vi "BallShear_BallShear_2.vi"(8 "Check":bool, 10 "Speed":dbl=2.0, 11 "Selected Balls":dbl[][](array[numeric])) -> (0 "Ready":bool, 2 "Waveform Stack":cluster{"Waveform Chart":dbl[]}[](array[cluster]) caption="Array of clusters, each containing one waveform chart")   [LabVIEW 2013]
panel:
  out "Status":string
  out "y":dbl
  out "x":dbl
  out "Selected Balls 2":dbl[](array[numeric])
  out "Z AFTER JOGGING":dbl
  in  "Waveform Chart":dbl(graph)
  out "Z Val":dbl
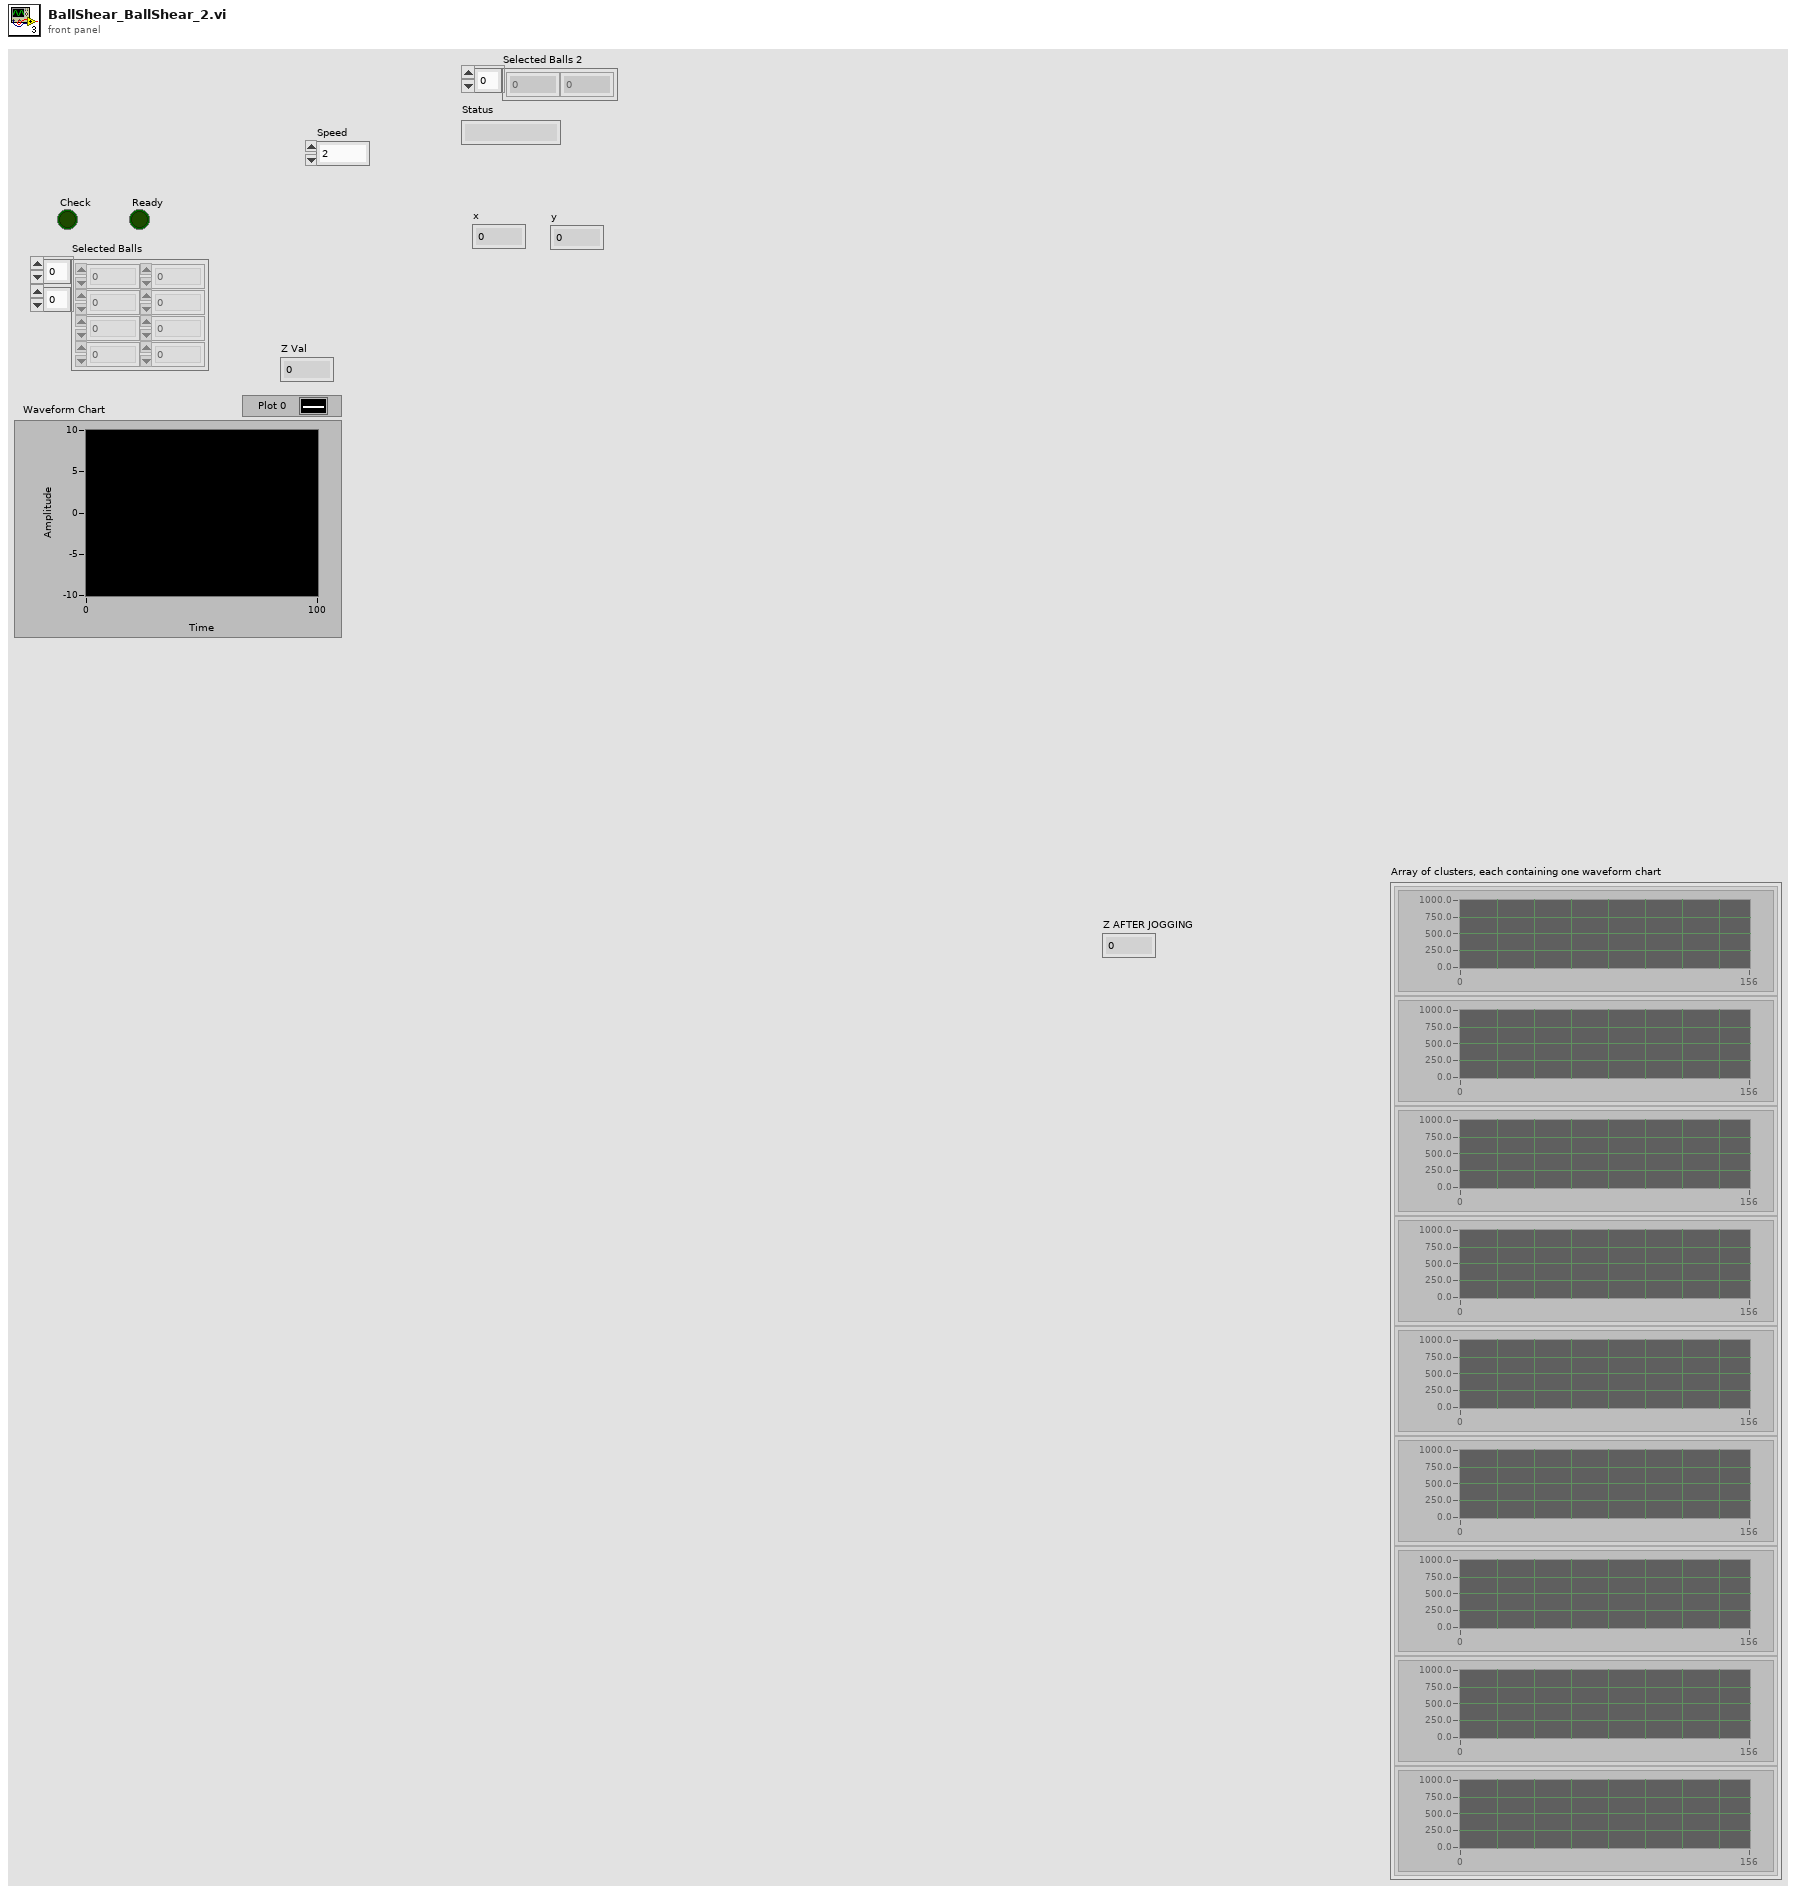
[diagram p1: front panel]
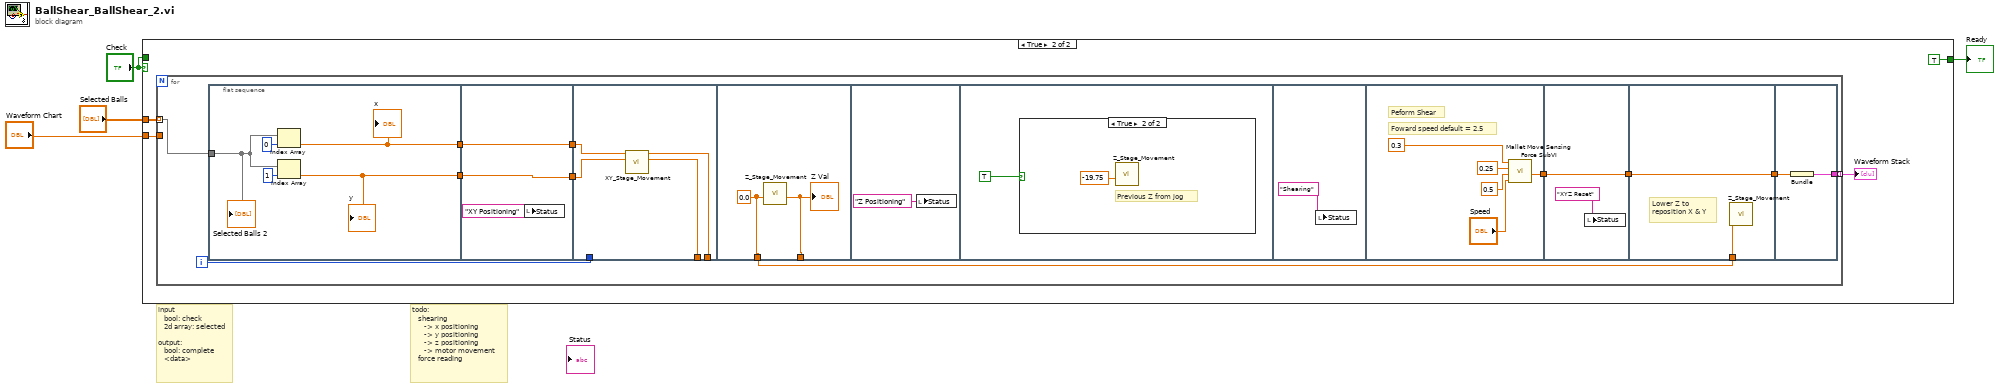
[diagram p0: block diagram]
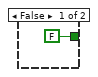
[diagram p2: hidden frame]
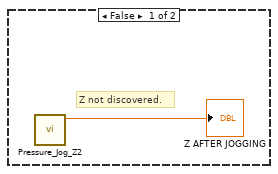
[diagram p3: hidden frame]
diagram:
  # "todo:\n   shearing\n      -> x positioning\n      -> y positioning\n      -> z positioning\n      -> motor movement\n   force reading"
  # "input\n   bool: check\n   2d array: selected\n\noutput:\n   bool: complete\n   <data>"
  n1 = case shown="True" "Check" {
    tunnel: "Check" -> [_ _]
    tunnel: [FALSE ("Power") TRUE ("Power")] -> w3
    tunnel: "Selected Balls" -> [_ w8]
    tunnel: "Waveform Chart" -> [_ w7]
    frame False {
    }
    frame True {
      n2 = for {
        tunnel: w8 -> [w16] mode=indexing
        tunnel: w7 -> [_]
        tunnel: [w19] -> w6 mode=indexing
        i -> [w20]
        n3 = flat-sequence {
          tunnel: w16 -> [w23]
          tunnel: [w22] -> w15
          tunnel: [w21] -> w13
          tunnel: w15 -> [w28]
          tunnel: [w28] -> w14
          tunnel: w13 -> [w27]
          tunnel: [w27] -> w12
          tunnel: w20 -> [_]
          tunnel: [w32] -> _
          tunnel: [w31] -> _
          tunnel: w14 -> [w30]
          tunnel: w12 -> [w29]
          tunnel: [w34] -> _
          tunnel: [w33] -> w17
          tunnel: [w40] -> w11
          tunnel: w11 -> [w46]
          tunnel: [w46] -> w10
          tunnel: w10 -> [w48]
          tunnel: [w48] -> w18
          tunnel: w17 -> [w47]
          tunnel: [w50] -> w19
          tunnel: w18 -> [w49]
          frame #0 {
            n4 = Index Array(array=w23, index=0) -> (element=w22:dbl)
            "x" <- w22
            n5 = Index Array(array=w23, index=1) -> (element=w21:dbl)
            "y" <- w21
            "Selected Balls 2" <- w23
          }
          frame #1 {
            n6 = local write "Status"("XY Positioning" ("Status")) -> ()
          }
          frame #2 {
            n7 = call "XY_Stage_Movement.vi"("Y Input"=w29, "X Input"=w30) -> ("Current Y Position"=w31:sgl, "Current X Position"=w32:sgl)  [unwired: 8 in]
          }
          frame #3 {
            w33 = 0.0 ("Z Input")
            n8 = call "Z_Stage_Movement.vi"("Z Input"=w33) -> ("Current Z Position"=w34:sgl)  [unwired: 10 in]
            "Z Val" <- w34
          }
          frame #4 {
            n9 = local write "Status"("Z Positioning" ("Status")) -> ()
          }
          frame #5 {
            n10 = case shown="True" TRUE {
              frame False {
                # "Z not discovered."
                n11 = call "Pressure_Jog_Z2.vi"() -> ("current Z"=→"Z AFTER JOGGING":sgl)  [unwired: 11 in]
              }
              frame True {
                # "Previous Z from jog"
                n12 = call "Z_Stage_Movement.vi"("Z Input"=-19.75) -> ()  [unwired: 10 in, 1 out]
              }
            }
          }
          frame #6 {
            n13 = local write "Status"("Shearing" ("Status")) -> ()
          }
          frame #7 {
            # "Foward speed default = 2.5"
            # "Peform Shear"
            n14 = call "Mallet Move Sensing Force SubVI.vi"("Forward Speed"="Speed", "Reverse Speed"=0.5, "Forward Time"=0.25, "Reverse Time"=0.3) -> ("Array of Forces"=w40:dbl[])  [unwired: 6 in, 1 out]
          }
          frame #8 {
            n15 = local write "Status"("XYZ Reset" ("Status")) -> ()
          }
          frame #9 {
            # "Lower Z to \nreposition X & Y"
            n16 = call "Z_Stage_Movement.vi"("Z Input"=w47) -> ()  [unwired: 10 in, 1 out]
          }
          frame #10 {
            n17 = Bundle("Array of Forces"=w49) -> (w50:cluster{"Array of Forces":dbl[]})  [unwired: 1 in]
          }
        }
      }
      "Waveform Stack" <- w6
    }
  }
  "Ready" <- w3
